vi "listSubclasses.vi"(11 "LabVIEW Object":refnum<class>) -> (0 "Subclasses objects":refnum<class>[](array[class]), 2 "Stripped subclasses names":string[](array[string]), 3 "Subclasses names":string[](array[string]))   [LabVIEW 2018]
uses:
  SupplyControl/SupplyControl.lvclass
panel:
  out "class name":string
  out "name":string
  out "stripped path":path
  out "All Files in Dir":path[](array[path])
  in  "SupplyControl.lvclass":refnum<class "SupplyControl.lvclass">
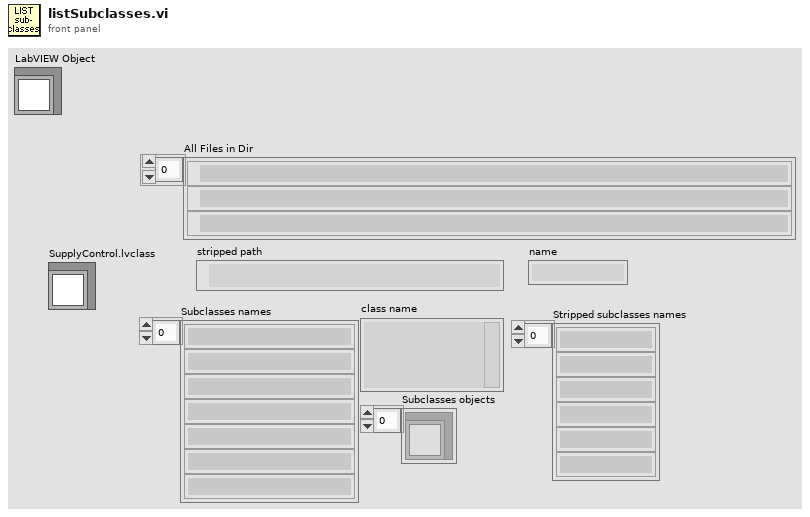
[diagram p1: front panel]
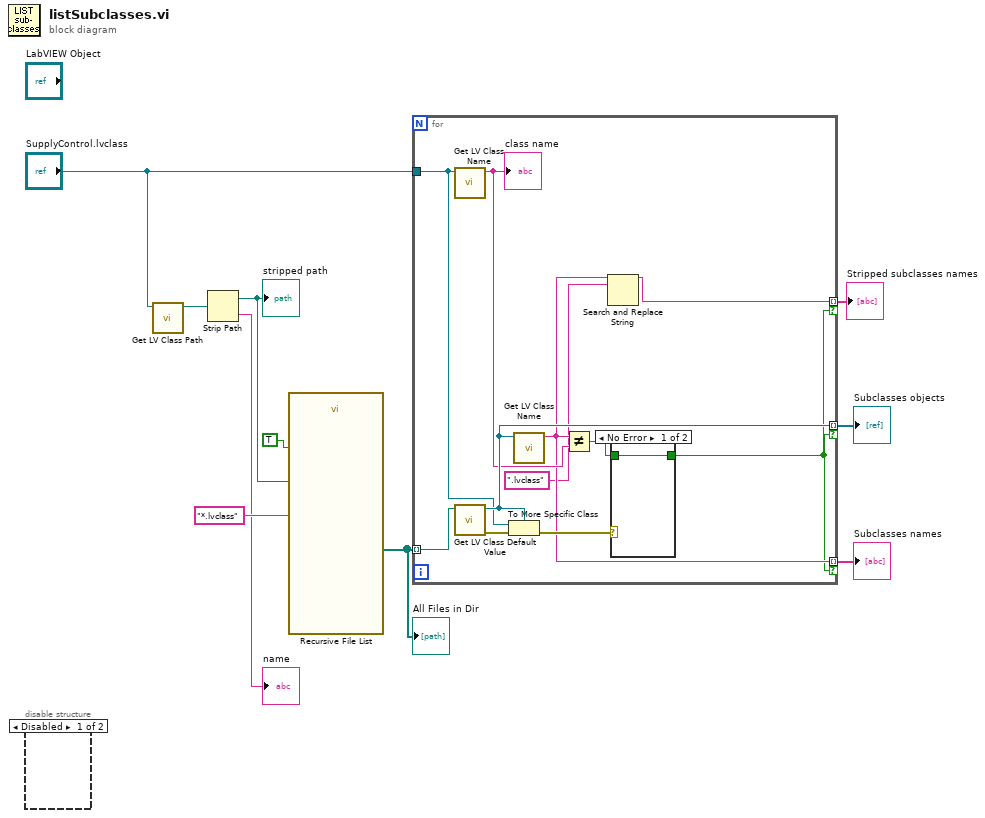
[diagram p0: block diagram]
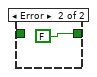
[diagram p3: hidden frame]
diagram:
  n1 = disable-structure shown="Disabled" {
    frame Disabled {
    }
    frame Enabled {
    }
  }
  n2 = call <vilib>:"Get LV Class Path.vi"("object"="SupplyControl.lvclass") -> ("class path"=w8:path)  [unwired: 9 in, 1 out]
  n3 = Strip Path(path=w8) -> (stripped path=w6:path, name=→"name":string)
  "stripped path" <- w6
  n4 = call <vilib>:"Recursive File List.vi"("pattern"="*.lvclass", "Continue Recursing on Error? (F)"=TRUE, "Folder Path"=w6) -> ("All Files in Dir"=w5:path[])  [unwired: 4 in, 4 out]
  "All Files in Dir" <- w5
  n5 = for {
    tunnel: w5 -> [w21] mode=indexing
    tunnel: "SupplyControl.lvclass" -> [w17]
    tunnel: [w18] -> w3 mode=indexing if=w11
    tunnel: [w14] -> w4 mode=indexing if=w11
    tunnel: [w12] -> w1 mode=indexing if=w11
    n6 = call <vilib>:"Get LV Class Name.vi"("object"=w17) -> ("class name"=w16:string)  [unwired: 9 in, 1 out]
    "class name" <- w16
    n7 = call <vilib>:"Get LV Class Default Value.vi"("class path"=w21) -> ("error out"=w20:errorcluster, "object"=w18:refnum<class>)  [unwired: 9 in]
    n8 = To More Specific Class(target class=w18, reference=w17, error in=w20) -> (error out=w19:errorcluster)  [unwired: 1 out]
    n9 = call <vilib>:"Get LV Class Name.vi"("object"=w18) -> ("class name"=w14:string)  [unwired: 9 in, 1 out]
    n10 = Not Equal?(x=w14, y=w16) -> (x != y?=w15:bool)
    n11 = Search and Replace String(input string=w14, search string=".lvclass" ("substring (\"\")")) -> (result string=w12:string)  [unwired: 6 in, 3 out]
    n12 = case shown="No Error" w19 {
      tunnel: [w22 FALSE] -> w11
      tunnel: w15 -> [w22 _]
      frame No Error {
      }
      frame Error {
      }
    }
  }
  "Subclasses names" <- w4
  "Subclasses objects" <- w3
  "Stripped subclasses names" <- w1
